vi "sv_UFF58 Check Data Valid (Time) (1Ch).vi"(5 "waveform":waveform(dbl)={"t0"=timestamp(0 s since 1904-01-01), "dt"=0.0, "Y"=[]}, 11 "error in (no error)":errorcluster) -> (6 "dup waveform":waveform(dbl), 15 "error out":errorcluster)   [LabVIEW 2017, in "SoundVib_UFF58.lvlib"]
doc: "This VI checks to see if the input waveform is empty"
uses:
  <vilib>/addons/Sound and Vibration/svt_UFF58/SoundVib_UFF58.lvlib
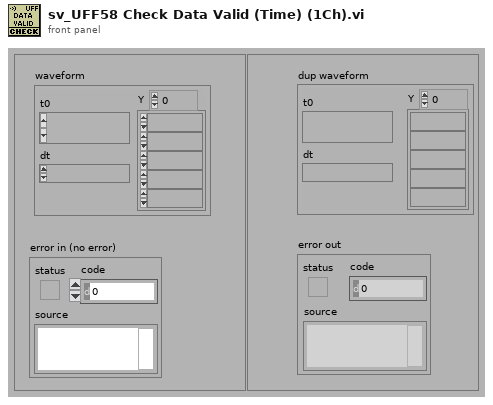
[diagram p1: front panel]
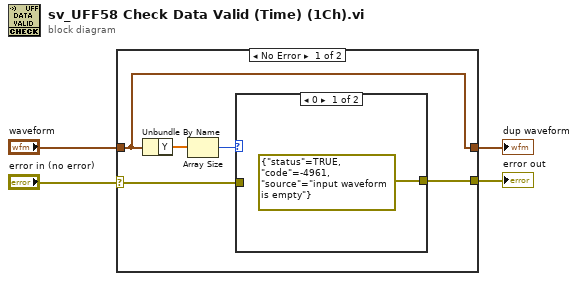
[diagram p0: block diagram]
diagram:
  n1 = case shown="No Error" "error in (no error)" {
    selector: "error in (no error)" -> [w7 w13]
    tunnel: "waveform" -> [w5 w12]
    tunnel: [w8 w13] -> w4
    tunnel: [w5 w12] -> w1
    frame No Error {
      n2 = Unbundle By Name(w5) -> ("Y"=w6:dbl[])
      n3 = Array Size(array=w6) -> (size(s)=w9:i32)
      n4 = case shown="0" w9 {
        tunnel: w7 -> [_ w11]
        tunnel: [errorcluster {"status"=TRUE, "code"=-4961, "source"="input waveform is empty"} ("error IO") w11] -> w8
        frame 0 {
        }
        frame 1, Default {
        }
      }
    }
    frame Error {
    }
  }
  "error out" <- w4
  "dup waveform" <- w1
